vi "indexing_steps.vi"(1 "z-score series (input)":dbl[](array[numeric])) -> (6 "index of step (output)":dbl[](array[numeric]))   [LabVIEW 2012]
uses:
  <vilib>/Analysis/baseanly.llb/Mean (DBL).vi
  <vilib>/Analysis/NI_AALBase.lvlib
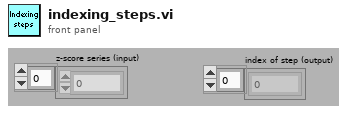
[diagram p1: front panel]
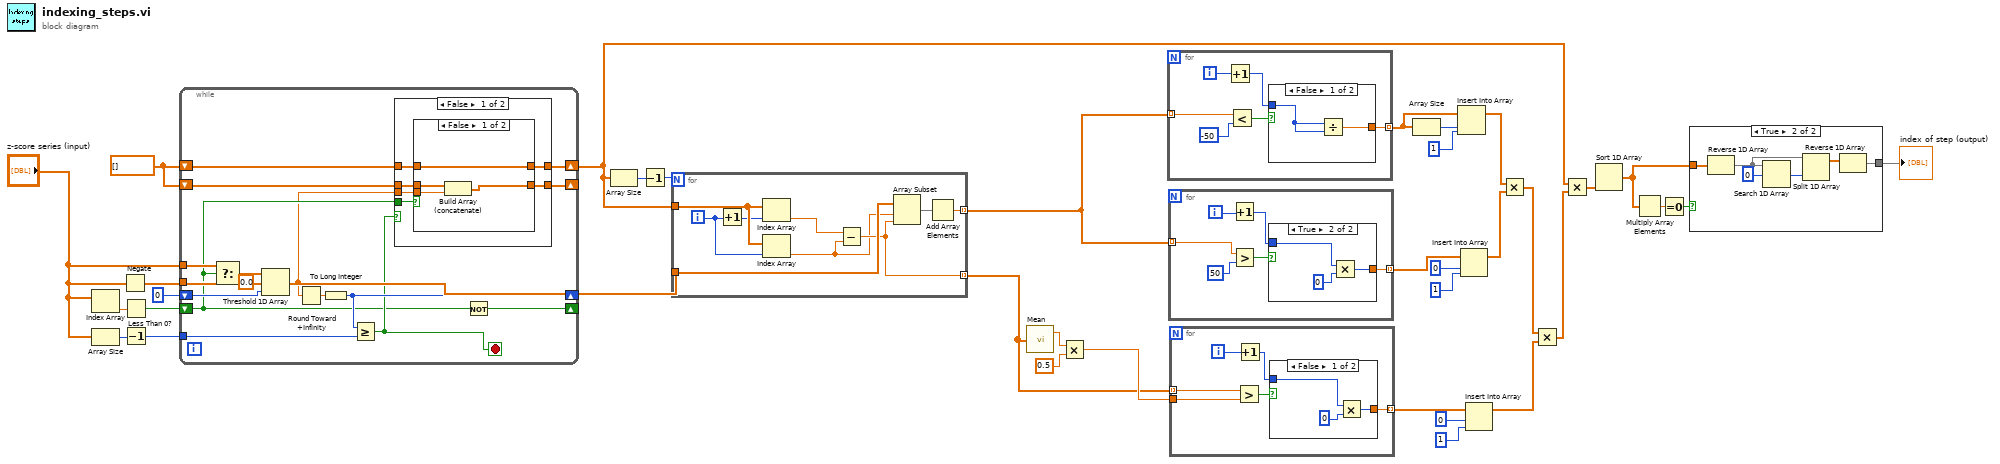
[diagram p0: block diagram]
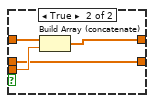
[diagram p2: hidden frame]
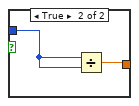
[diagram p5: hidden frame]
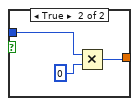
[diagram p6: hidden frame]
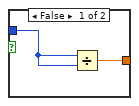
[diagram p7: hidden frame]
diagram:
  w27 = dbl[] []
  n1 = Index Array(array="z-score series (input)") -> (element=w32:dbl)  [unwired: 1 in]
  n2 = Array Size(array="z-score series (input)") -> (size(s)=w29:i32)
  n3 = Negate(x="z-score series (input)") -> (-x=w33:dbl[])
  n4 = Less Than 0?(x=w32) -> (x < 0?=w31:bool)
  n5 = Decrement(x=w29) -> (x-1=w28:i32)
  n6 = while {
    tunnel: "z-score series (input)" -> [w51]
    tunnel: w33 -> [w50]
    shift-right: [w46] -> _
    shift-left: w31 -> [w41]
    shift-right: [w44] -> _
    shift-left: 0 -> [w47]
    shift-right: [w38] -> w35
    shift-left: w27 -> [w40]
    shift-right: [w36] -> _
    shift-left: w27 -> [w37]
    tunnel: w28 -> [w43]
    stop <- w42 stop-if-true
    n7 = Select(t=w51, s=w41, f=w50) -> (s? t:f=w49:dbl[])
    n8 = Threshold 1D Array(1:w47, 2:0.0 ("threshold y"), 3:w49) -> (0:w39:dbl)
    n9 = Round Toward +Infinity(x=w39) -> (ceil(x): smallest int >= x=w45:dbl)
    n10 = To Long Integer(number=w45) -> (32bit integer=w44:i32)
    n11 = Greater Or Equal?(x=w44, y=w43) -> (x >= y?=w42:bool)
    n12 = case shown="False" w42 {
      tunnel: w41 -> [w57 _]
      tunnel: w40 -> [w56 w67]
      tunnel: w39 -> [w55 _]
      tunnel: [w54 w67] -> w38
      tunnel: w37 -> [w53 w66]
      tunnel: [w52 w66] -> w36
      frame False {
        n13 = case shown="False" w57 {
          tunnel: w56 -> [w61 w65]
          tunnel: w55 -> [w58 w64]
          tunnel: [w61 w63] -> w54
          tunnel: w53 -> [w60 w62]
          tunnel: [w59 w62] -> w52
          frame False {
            n14 = Build Array (concatenate)(w60, w58) -> (w59:dbl[])
          }
          frame True {
            n15 = Build Array (concatenate)(w65, w64) -> (w63:dbl[])
          }
        }
      }
      frame True {
      }
    }
    n16 = Not(x=w41) -> (.not. x?=w46:bool)
  }
  n17 = Array Size(array=w35) -> (size(s)=w2:i32)
  n18 = Decrement(x=w2) -> (x-1=w1:i32)
  n19 = for {
    N: w1 -> [_]
    tunnel: w35 -> [w76]
    tunnel: "z-score series (input)" -> [w73]
    tunnel: [w71] -> w3 mode=indexing
    tunnel: [w70] -> w14 mode=indexing
    i -> [w74]
    n20 = Increment(x=w74) -> (x+1=w75:i32)
    n21 = Index Array(array=w76, index=w75) -> (element=w69:dbl)
    n22 = Index Array(array=w76, index=w74) -> (element=w68:dbl)
    n23 = Subtract(x=w69, y=w68) -> (x-y=w70:dbl)
    n24 = Array Subset(array=w73, index=w68, length=w70) -> (w72:dbl[])
    n25 = Add Array Elements(numeric array=w72) -> (sum=w71:dbl)
  }
  n26 = call-poly <vilib>:"Mean.vi"("X"=w14) -> ("mean"=w12:dbl)  [unwired: 1 out]
  n27 = Multiply(x=w12, y=0.5) -> (x*y=w15:dbl)
  n28 = for {
    tunnel: w3 -> [w79] mode=indexing
    tunnel: [w77] -> w5 mode=indexing
    i -> [w82]
    n29 = Increment(x=w82) -> (x+1=w78:i32)
    n30 = Less?(x=w79, y=-50) -> (x < y?=w81:bool)
    n31 = case shown="False" w81 {
      tunnel: w78 -> [w84 w86]
      tunnel: [w83 w85] -> w77
      frame False {
        n32 = Divide(x=w84, y=w84) -> (x/y=w83:dbl)
      }
      frame True {
        n33 = Multiply(x=w86, y=0) -> (x*y=w85:i32)
      }
    }
  }
  n34 = for {
    tunnel: w3 -> [w91] mode=indexing
    tunnel: [w88] -> w9 mode=indexing
    i -> [w90]
    n35 = Increment(x=w90) -> (x+1=w89:i32)
    n36 = Greater?(x=w91, y=50) -> (0:w93:bool)
    n37 = case shown="True" w93 {
      tunnel: w89 -> [w94 w97]
      tunnel: [w95 w96] -> w88
      frame False {
        n38 = Divide(x=w94, y=w94) -> (x/y=w95:dbl)
      }
      frame True {
        n39 = Multiply(x=w97, y=0) -> (x*y=w96:i32)
      }
    }
  }
  n40 = for {
    tunnel: w14 -> [w101] mode=indexing
    tunnel: w15 -> [w100]
    tunnel: [w99] -> w18 mode=indexing
    i -> [w104]
    n41 = Greater?(x=w101, y=w100) -> (0:w102:bool)
    n42 = Increment(x=w104) -> (x+1=w103:i32)
    n43 = case shown="False" w102 {
      tunnel: w103 -> [w106 w109]
      tunnel: [w105 w108] -> w99
      frame False {
        n44 = Multiply(x=w106, y=0) -> (x*y=w105:i32)
      }
      frame True {
        n45 = Divide(x=w109, y=w109) -> (x/y=w108:dbl)
      }
    }
  }
  n46 = Array Size(array=w5) -> (size(s)=w4:i32)
  n47 = Insert Into Array(array=w5, index=w4, new element=1) -> (w10:dbl[])
  n48 = Insert Into Array(array=w9, index=0, new element=1) -> (w11:dbl[])
  n49 = Insert Into Array(array=w18, index=0, new element=1) -> (w20:dbl[])
  n50 = Multiply(x=w10, y=w11) -> (x*y=w19:dbl[])
  n51 = Multiply(x=w19, y=w20) -> (x*y=w21:dbl[])
  n52 = Multiply(x=w35, y=w21) -> (x*y=w22:dbl[])
  n53 = Sort 1D Array(array=w22) -> (sorted array=w25:dbl[])
  n54 = Multiply Array Elements(1:w25) -> (0:w23:dbl)
  n55 = Equal To 0?(x=w23) -> (x = 0?=w24:bool)
  n56 = case shown="True" w24 {
    tunnel: w25 -> [w110 w116]
    tunnel: [w110 w111] -> w26
    frame False {
    }
    frame True {
      n57 = Reverse 1D Array(array=w116) -> (reversed array=w113:dbl[])
      n58 = Search 1D Array(1D array=w113, element=0) -> (index of element=w114:i32)  [unwired: 1 in]
      n59 = Split 1D Array(array=w113, index=w114) -> (first subarray=w112:dbl[])  [unwired: 1 out]
      n60 = Reverse 1D Array(array=w112) -> (reversed array=w111:dbl[])
    }
  }
  "index of step (output)" <- w26
